vi "testing_wfm-string_to_LV-array.vi"() -> ()   [LabVIEW 2019, in "mmW_commands.lvlib"]
uses:
  mmW_commands.lvlib
  <vilib>/measure/maspectr.llb/FFT Power Spectrum and PSD for 1 Chan (CDB).vi
  <vilib>/measure/NI_MAPro.lvlib
panel:
  out "Power Spectrum / PSD":cluster{"f0":dbl, "df":dbl, "magnitude":dbl[]}(graph)
  out "Graph 2":dbl[][](graph)
  out "Interleaved graph":dbl[](graph)
  out "Interleaved data":dbl[](array[numeric])
  out "Data size (B)":i32
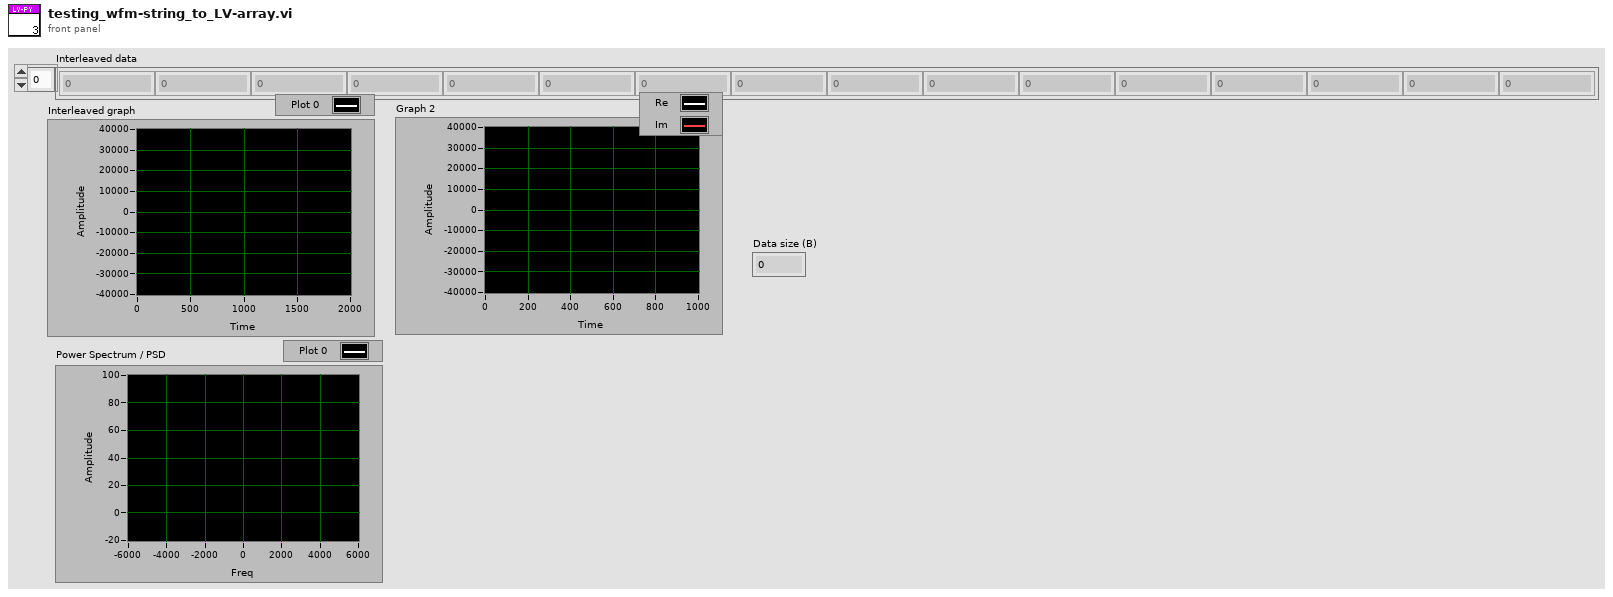
[diagram p1: front panel]
types:
  T1 = enum16{"numpy.ndarray, int32", "numpy.ndarray,int16"}
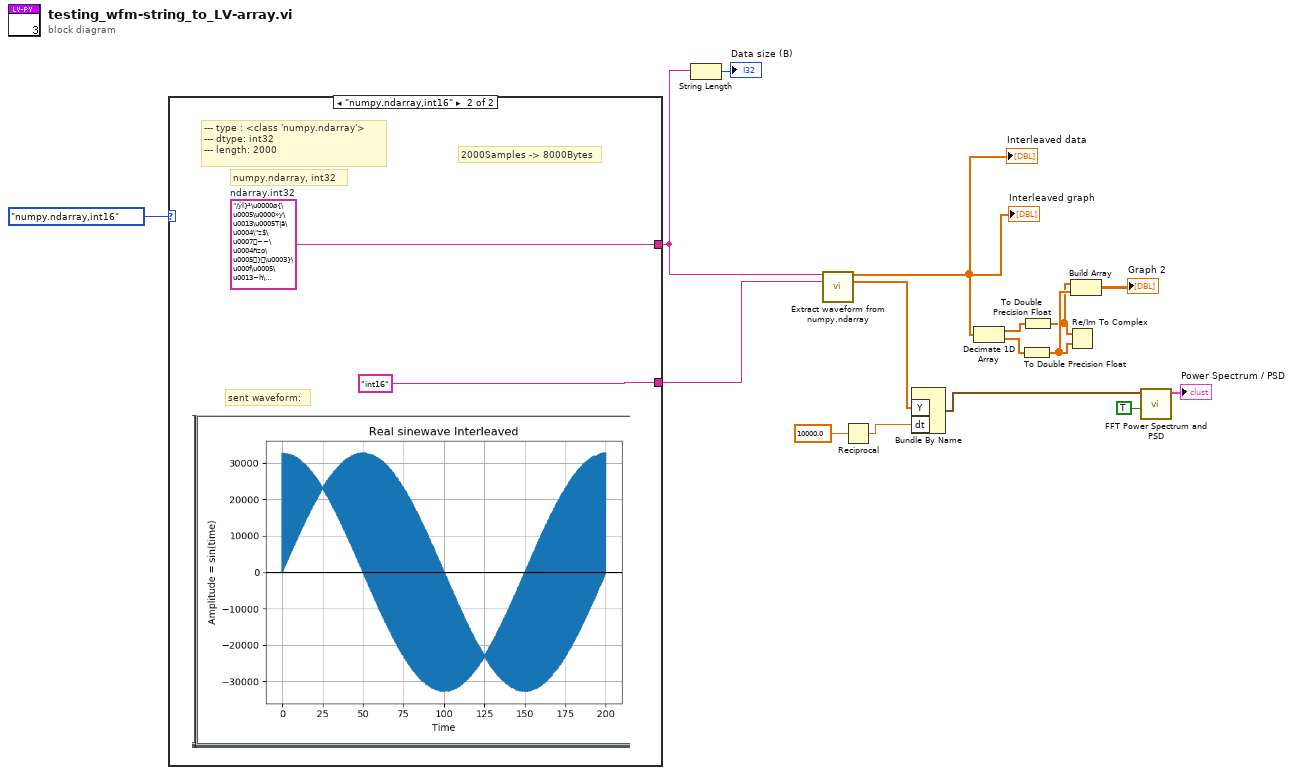
[diagram p0: block diagram]
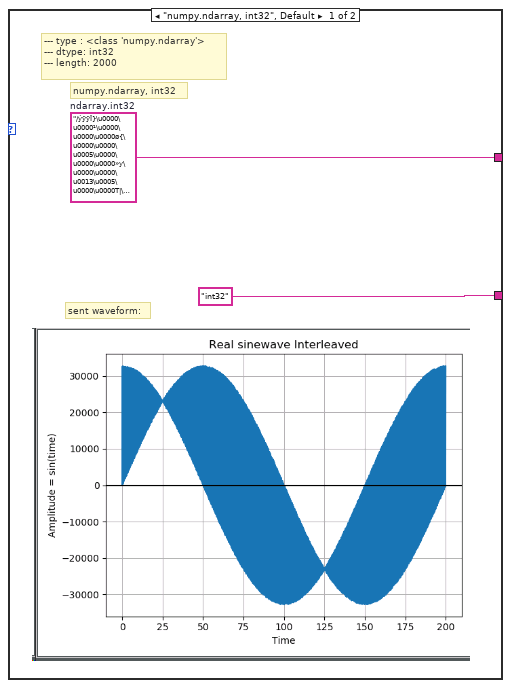
[diagram p2: hidden frame]
diagram:
  n1 = case shown="\"numpy.ndarray,int16\"" T1."numpy.ndarray,int16" {
    tunnel: [w18 w20] -> w14
    tunnel: ["int32" "int16"] -> w13
    frame "numpy.ndarray, int32", Default {
      w18 = "/ýÿÿÎ}\u0000\u0000¹\u0000\u0000\u0000ø{\u0000\u0000\u0005\u0000\u0000\u0000»y\u0000\u0000\u0013\u0005\u0000\u0000T|\u0000\u0000ä\u0004\u0000\u0000\"z\u0000\u0000$\u0007\u0000\u0000~\u0000\u0000~\u0004\u0000\u0000ñz\u0000\u0000o\u0005\u0000\u0000}\u0000\u0000\u0003\u0000\u0000}\u0000\u0000\u000f\u0005\u0000\u0000\u0013~\u0000\u0000h\u000b\u0000\u0000y\u0000\u0000)\u0006\u0000\u0000»|\u0000\u0000\b\u0000\u0000x\u0000\u0000N\u0007\u0000\u0000\u0010}\u0000\u0000¤\n\u0000\u0000÷~\u0000\u0000F\n\u0000\u0000x\u0000\u0000Ð\r\u0000\u0000\u0014\u0000\u0000@\u0010\u0000\u0000vz\u0000\u0000­\n\u0000\u00000|\u0000\u0000¹\u000f\u0000\u0000¸z\u0000\u0000ÿ\r\u0000\u0000ëz\u0000\u0000\u0016\u0010\u0000\u0000*}\u0000\u0000)\u0011\u0000\u0000{\u0000\u0000\u000e\u0000\u0000¤~\u0000\u0000ì\u0010\u0000\u0000¨{\u0000\u0000e\u0013\u0000\u0000.z\u0000\u0000\u000e\u0012\u0000\u0000f}\u0000\u0000\u0013\u0000\u0000\"x\u0000\u0000.\u0014\u0000\u0000Pw\u0000\u0000÷\u0014\u0000\u0000[w\u0000\u0000¿\u0013\u0000\u0000³z\u0000\u0000£\u0018\u0000\u0000©{\u0000\u0000ó\u0018\u0000\u0000v\u0000\u0000¥\u001c\u0000\u0000é|\u0000\u0000m\u001b\u0000\u0000/w\u0000\u0000\u0019\u0000\u0000¤y\u0000\u0000¥\u0019\u0000\u0000¸{\u0000\u0000\"\u001d\u0000\u0000sx\u0000\u0000i \u0000\u0000u\u0000\u0000é\u001e\u0000\u0000»u\u0000\u0000¤\"\u0000\u0000Yx\u0000\u0000Þ \u0000\u0000ü{\u0000\u0000\"\u0000\u0000µw\u0000\u0000\u000b#\u0000\u0000·w\u0000\u0000j\u001e\u0000\u0000:z\u0000\u0000v$\u0000\u0000»x\u0000\u0000\t!\u0000\u00003u\u0000\u0000Ð'\u0000\u0000Ww\u0000\u0000ü\"\u0000\u0000qv\u0000\u0000N\"\u0000\u0000t\u0000\u0000s&\u0000\u0000?v\u0000\u0000Î*\u0000\u0000¢y\u0000\u0000ø'\u0000\u0000üx\u0000\u0000ø*\u0000\u0000ðs\u0000\u0000u,\u0000\u0000¿w\u0000\u0000p&\u0000\u0000^r\u0000\u0000)\u0000\u0000Ör\u0000\u0000ª+\u0000\u0000xu\u0000\u0000R*\u0000\u0000Þt\u0000\u0000²-\u0000\u0000)u\u0000\u0000/\u0000\u0000ìp\u0000\u0000N-\u0000\u0000ão\u0000\u0000:.\u0000\u0000)u\u0000\u0000­3\u0000\u0000Vv\u0000\u0000X-\u0000\u0000\u0000t\u0000\u0000\u00024\u0000\u0000ªs\u0000\u0000¢2\u0000\u0000lr\u0000\u0000\r6\u0000\u0000js\u0000\u0000â4\u0000\u0000tn\u0000\u00001\u0000\u0000q\u0000\u0000Ä6\u0000\u0000îm\u0000\u0000»5\u0000\u0000Ãn\u0000\u0000ý6\u0000\u0000ql\u0000\u0000\\9\u0000\u0000³p\u0000\u0000:\u0000\u0000èq\u0000\u0000..."  # ndarray.int32
      # "sent waveform:"
      # "numpy.ndarray, int32"
      # "--- type : <class 'numpy.ndarray'>\n--- dtype: int32\n--- length: 2000"
    }
    frame "numpy.ndarray,int16" {
      w20 = "/ýÎ}¹\u0000ø{\u0005\u0000»y\u0013\u0005T|ä\u0004\"z$\u0007~~\u0004ñzo\u0005}\u0003}\u000f\u0005\u0013~h\u000by)\u0006»|\bxN\u0007\u0010}¤\n÷~F\nxÐ\r\u0014@\u0010vz­\n0|¹\u000f¸zÿ\rëz\u0016\u0010*})\u0011{\u000e¤~ì\u0010¨{e\u0013.z\u000e\u0012f}\u0013\"x.\u0014Pw÷\u0014[w¿\u0013³z£\u0018©{ó\u0018v¥\u001cé|m\u001b/w\u0019¤y¥\u0019¸{\"\u001dsxi ué\u001e»u¤\"YxÞ ü{\"µw\u000b#·wj\u001e:zv$»x\t!3uÐ'Wwü\"qvN\"ts&?vÎ*¢yø'üxø*ðsu,¿wp&^r)Örª+xuR*Þt²-)u/ìpN-ão:.)u­3VvX-\u0000t\u00024ªs¢2lr\r6jsâ4tn1qÄ6îm»5Ãný6ql\\9³p:èq;Zo´9£p³<j=Äp38\u001alµ8ik²<Ói#=úh\u0013AQh¸=6hâ?g>@Lk*>Ñjõ=}j§B\bmÒEfÂCSeßBÝeõCºj\u0007EçikGxe\u0000C\u0000gD9fÍF2c8Kòc¤HÂaåFºeKI}a\u001bK\u000ecvK3e\nLª`IÇa\tM5d\fN\u0004^ÑO÷_QÍa\u001eOë^KN a¾RÉa\u000bOÖ]yQX]\u000eUCZgPa^kU\\eWNYèSZ\u0014XY\u0015U8[LZIX [ñ[³X\u0001YÌV\nU[\u0002Y:W\fTÌV6TWêUçWGRn]\u000fS3Z@TZðT®`ÛR!^P¯[ÐSA\\bQÐ\\VRJ]òK¹cûM6]öOí`XMdK7`H``K¿eþKæf¯FÿcNK..."  # ndarray.int32
      # "2000Samples -> 8000Bytes"
      # "sent waveform:"
      # "numpy.ndarray, int32"
      # "--- type : <class 'numpy.ndarray'>\n--- dtype: int32\n--- length: 2000"
    }
  }
  n2 = String Length(string=w14) -> (length=→"Data size (B)":i32)
  n3 = call "Extract waveform from numpy.ndarray.vi"("flattened data"=w14, 5:w13) -> ("Interleaved array"=w8:dbl[], "Complex array"=w6:cdb[])  [unwired: 12 in]
  "Interleaved data" <- w8
  "Interleaved graph" <- w8
  n4 = Reciprocal(x=10000.0) -> (1/x=w4:dbl)
  n5 = Bundle By Name("Y"=w6, "dt"=w4) -> (w3:waveform(cdb))  [unwired: 1 in]
  n6 = Decimate 1D Array(w8) -> (w9:dbl[], w10:dbl[])
  n7 = To Double Precision Float(number=w10) -> (double precision float=w12:dbl[])
  n8 = To Double Precision Float(number=w9) -> (double precision float=w11:dbl[])
  n9 = Re/Im To Complex(1:w12, 2:w11) -> ()  [unwired: 1 out]
  n10 = Build Array(w11, w12) -> (→"Graph 2":dbl[][])
  n11 = call-poly <vilib>:"FFT Power Spectrum and PSD.vi"("dB On (F)"=TRUE, "time signal"=w3) -> ("Power Spectrum / PSD"=→"Power Spectrum / PSD":cluster{"f0":dbl, "df":dbl, "magnitude":dbl[]})  [unwired: 6 in, 3 out]
